vi "Incriment.vi"(8 "error in (no error)":errorcluster, 11 "Test-Client in":refnum<class "Test-Client.lvclass">) -> (0 "error out":errorcluster, 3 "Test-Client out":refnum<class "Test-Client.lvclass">)   [LabVIEW 2020, in "Test-Client.lvlib" / "Test-Client.lvclass"]
uses:
  Test-Client.lvclass
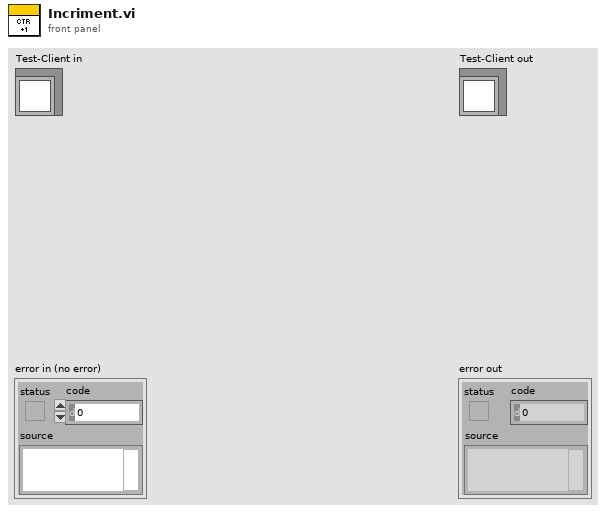
[diagram p1: front panel]
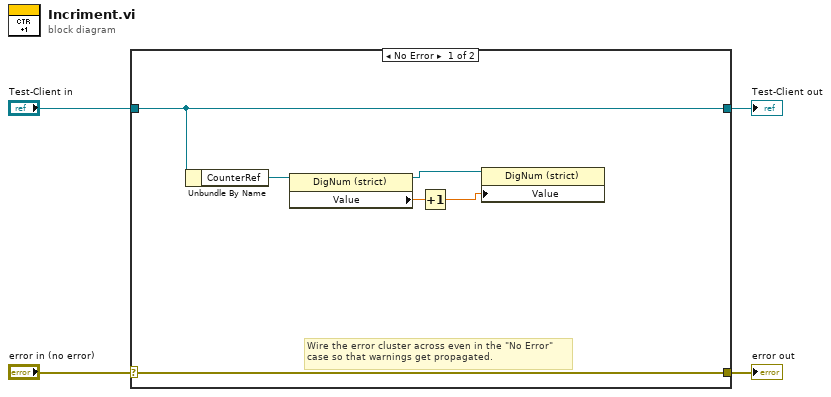
[diagram p0: block diagram]
diagram:
  n1 = case shown="No Error" "error in (no error)" {
    selector: "error in (no error)" -> [w10 w12]
    tunnel: [w10 w12] -> w3
    tunnel: [w9 w11] -> w1
    tunnel: "Test-Client in" -> [w9 w11]
    frame No Error {
      # "Wire the error cluster across even in the \"No Error\"\ncase so that warnings get propagated."
      n2 = Unbundle By Name(w9) -> ("CounterRef"=w8:refnum<vi>)
      n3 = property class="DigNum (strict)"(reference=w8) -> (reference out=w7:refnum<vi>, "Value"=w6:dbl)  [unwired: 1 in, 1 out]
      n4 = Increment(x=w6) -> (x+1=w5:dbl)
      n5 = property class="DigNum (strict)"(reference=w7, "Value"=w5) -> ()  [unwired: 1 in, 2 out]
    }
    frame Error {
    }
  }
  "error out" <- w3
  "Test-Client out" <- w1
